vi "MultiRun Description.vi"(11 "Send Emails?":bool=TRUE) -> (3 "Send Emails? Out":bool=TRUE)   [LabVIEW 2022 SP3]
uses:
  File/Setup_Filetype.ctl
  ADAM Client/Sub VIs/ADAM Controls/Module_type_ADAM.ctl
  ADAM Client/Sub VIs/ADAM Controls/Update_scan_value.ctl
  ADAM Client/Sub VIs/ADAM Controls/Calib_type_ADAM.ctl
  ADAM Client/Sub VIs/ADAM Controls/Channel_State.ctl
  <vilib>/Utility/error.llb/Trim Whitespace One-Sided.vi
  Globals/Constants_global.vi
  Globals/Preference_global.vi
  Globals/Trav_pos_global.vi
panel:
  in  "Stop":bool
  in  "Increment Run Number":bool=TRUE
  out "Results File Prefix":string
  in  "Project":u16(ring) items=["Add New Project", "G142-3D", "G142-3D"]
  in  "OK":bool
  out "Channel Name":string
  in  "Previous Messages:":u16(ring) items=["test"]
  in  "Please add a Multi Run Description:":string
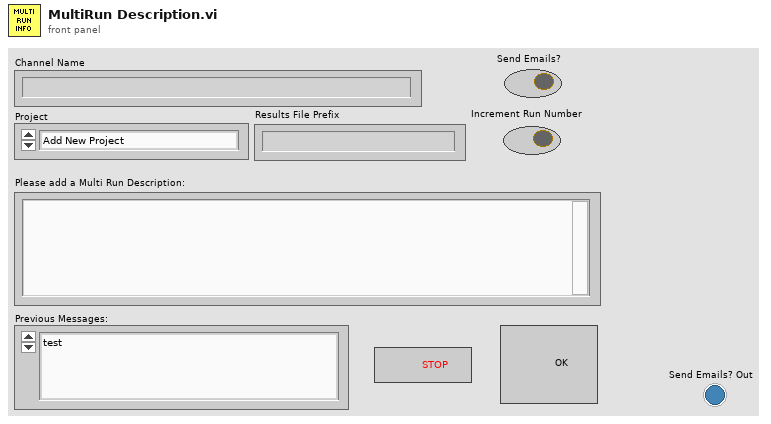
[diagram p1: front panel]
types:
  T1 = typedef "Setup_Filetype.ctl" = enum16{"Measurement Setups", "Calibration Setups", "General", "Results File Plotter Setups", "Speed Calib Tweaks"}
  T2 = typedef "Channel_State.ctl" = enum16{"On", "Off", "Always On", "Always Off"}
  T3 = typedef "Update_scan_value.ctl" = cluster{"Channel Name":string, "New Value":dbl, "!Auto_Off":bool}
  T4 = typedef "Module_type_ADAM.ctl" = string
  T5 = typedef "Ch_description_ADAM.ctl" = cluster{"Ch Name":string, "Type":T4, "Function":T6, "Ch State":T2, "Calibration type":T7, "A":dbl, "B":dbl, "C":dbl, "D":dbl, "Comments":string, "Address":T8, "String":string, "Duty":u16}
  T6 = typedef "Function_ADAM.ctl" = enum16{"Analogue Input", "Digital Input", "Event counter", "Event rate", "Analogue Output", "Digital Output", "Relay Output"}
  T7 = typedef "Calib_type_ADAM.ctl" = string
  T8 = typedef "Address.ctl" = cluster{"Main":i32, "Ch.":i32, "Sub":i32, "Port Name":string}
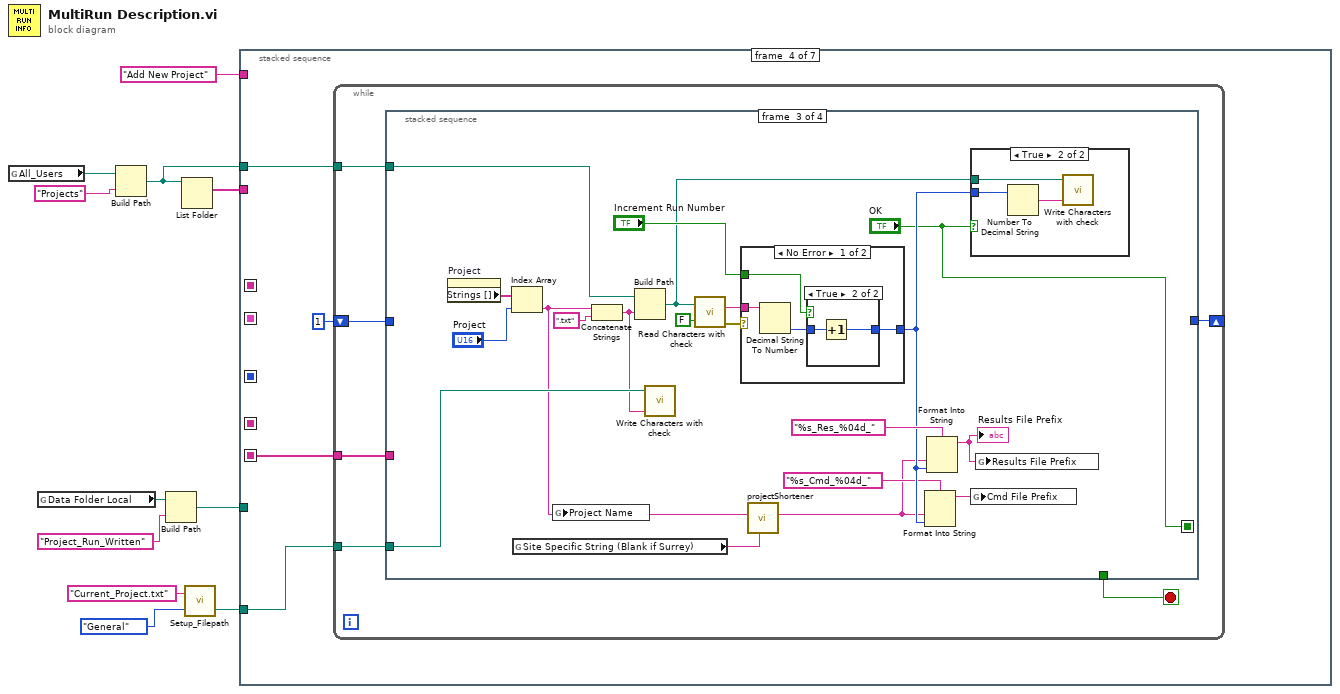
[diagram p0: block diagram]
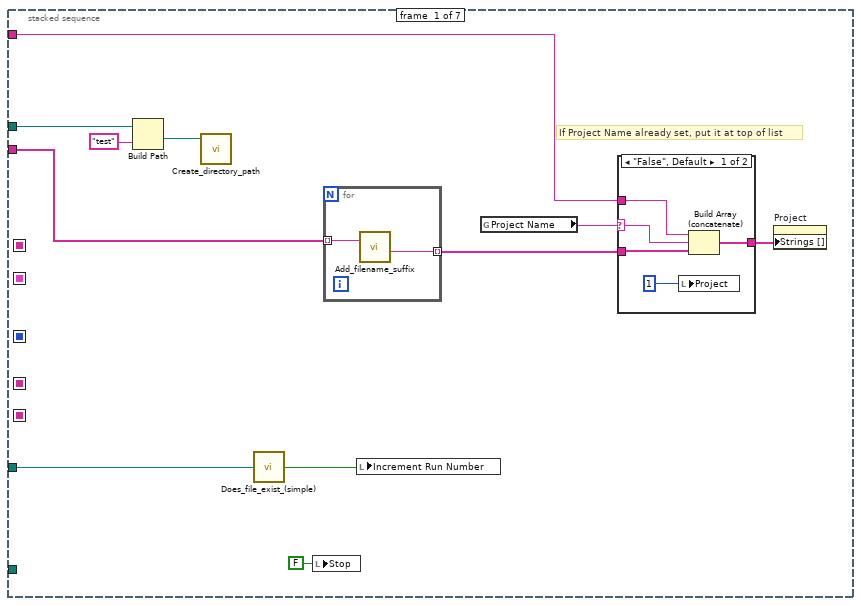
[diagram p2: hidden frame]
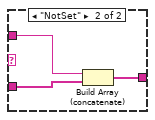
[diagram p3: hidden frame]
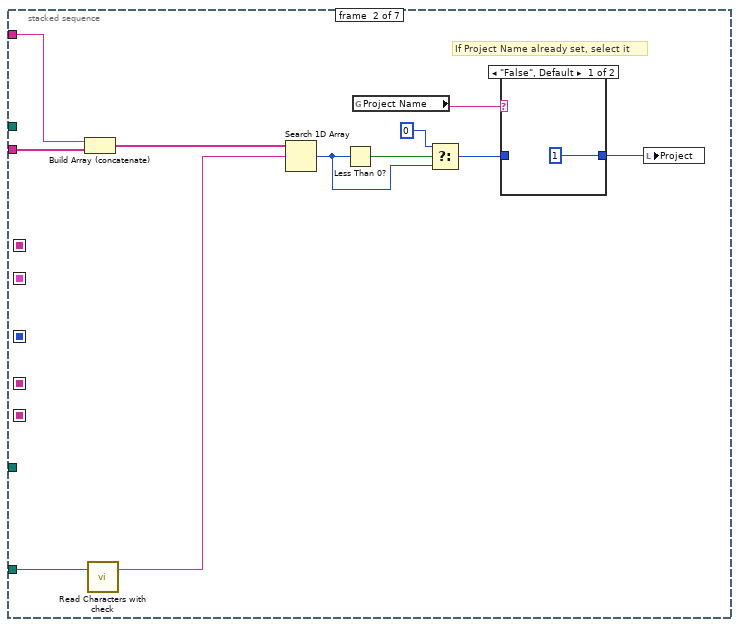
[diagram p4: hidden frame]
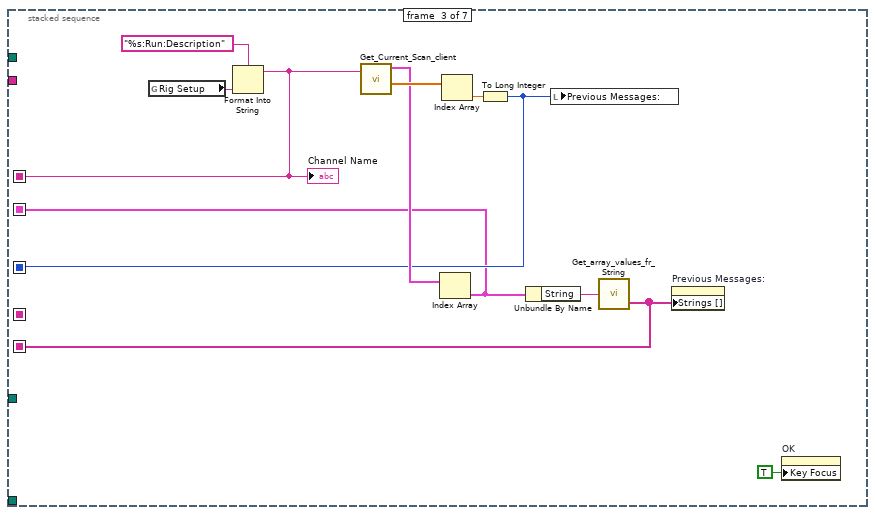
[diagram p6: hidden frame]
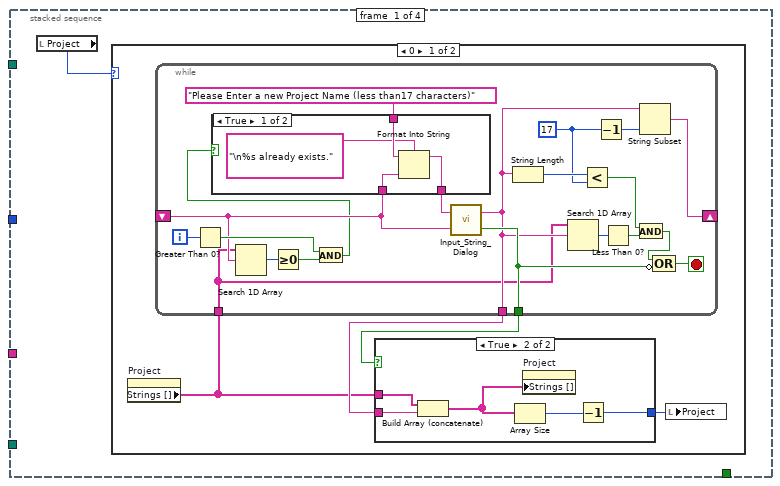
[diagram p7: hidden frame]
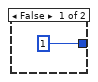
[diagram p8: hidden frame]
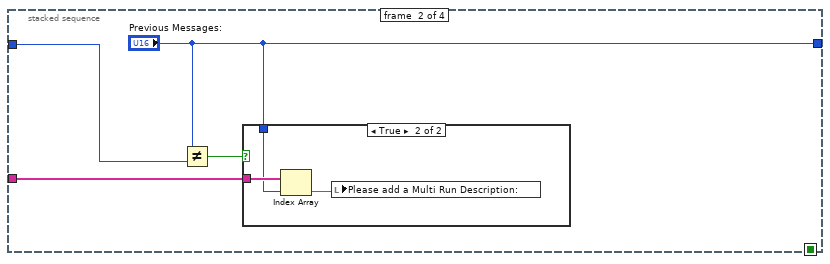
[diagram p11: hidden frame]
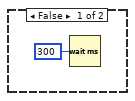
[diagram p12: hidden frame]
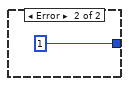
[diagram p15: hidden frame]
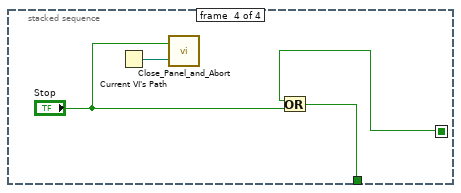
[diagram p16: hidden frame]
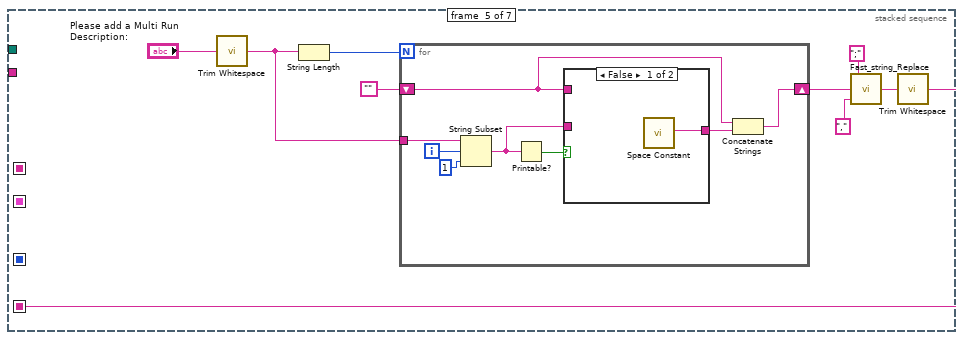
[diagram p17: hidden frame]
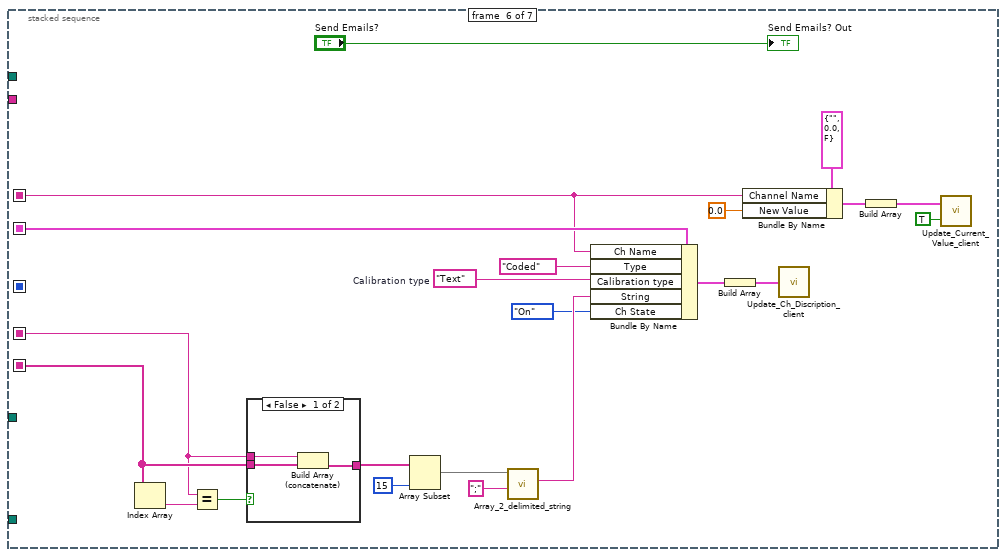
[diagram p19: hidden frame]
diagram:
  n1 = global read "Constants_global.vi" "All_Users"() -> (w8:path)
  n2 = global read "Constants_global.vi" "Data Folder Local"() -> (w3:path)
  n3 = Build Path(base path=w8, name or relative path="Projects") -> (appended path=w5:path)
  n4 = Build Path(base path=w3, name or relative path="Project_Run_Written") -> (appended path=w1:path)
  n5 = List Folder(path=w5) -> (filenames=w6:string[])  [unwired: 3 in, 3 out]
  n6 = call "Setup_Filepath.vi"("Setup File Type"=Setup_Filetype."General", "Filename in"="Current_Project.txt") -> ("Filename Out"=w9:path)  [unwired: 1 out]
  n7 = stacked-sequence {
    seq-local: [_ _ w51 _ _ _ _] -> [_ _ _ w60 _ w174 _]
    seq-local: [_ _ w49 _ _ _ _] -> [_ _ _ _ _ _ _]
    seq-local: [_ _ w48 _ _ _ _] -> [_ _ _ _ _ w186 _]
    seq-local: [_ _ w47 _ _ _ _] -> [_ _ _ _ _ w178 _]
    seq-local: [_ _ _ _ w146 _ _] -> [_ _ _ _ _ w167 _]
    tunnel: w9 -> [_ w34 _ w57 _ _ _]
    tunnel: w6 -> [w22 w40 _ _ _ _ _]
    tunnel: w5 -> [w20 _ _ w58 _ _ _]
    tunnel: "Add New Project" ("Base name") -> [w13 w41 _ _ _ _ _]
    tunnel: w1 -> [w15 _ _ _ _ _ w191]
    frame #0 {
      # "If Project Name already set, put it at top of list"
      n8 = Build Path(base path=w20, name or relative path="test") -> (appended path=w18:path)
      n9 = call "Create_directory_path.vi"("Path name"=w18) -> ()  [unwired: 2 in, 2 out]
      n10 = call "Does_file_exist_(simple).vi"("Pathname"=w15) -> ("exists?"=w16:bool)
      n11 = local write "Stop"(FALSE ("Stop")) -> ()
      n12 = for {
        tunnel: w22 -> [w32] mode=indexing
        tunnel: [w31] -> w21 mode=indexing
        n13 = call "Add_filename_suffix.vi"("Filename"=w32) -> ("Base name"=w31:string)  [unwired: 1 in, 3 out]
      }
      n14 = local write "Increment Run Number"(w16) -> ()
      n15 = global read "Preference_global.vi" "Project Name"() -> (w14:string)
      n16 = case shown="\"False\", Default" w14 {
        selector: w14 -> [w26 _]
        tunnel: w21 -> [w27 w30]
        tunnel: [w24 w29] -> w12
        tunnel: w13 -> [w25 w28]
        frame "False", Default {
          n17 = local write "Project"(1) -> ()
          n18 = Build Array (concatenate)(w25, w26, w27) -> (w24:string[])
        }
        frame "NotSet" {
          n19 = Build Array (concatenate)(w28, w30) -> (w29:string[])
        }
      }
      n20 = property on="Project" class="Ring (strict)"("Strings []"=w12) -> ()  [unwired: 2 in, 2 out]
    }
    frame #1 {
      # "If Project Name already set, select it"
      n21 = Build Array (concatenate)(w41, w40) -> (w39:string[])
      n22 = call "Read Characters with check.vi"("file (use dialog)"=w34) -> ("Read String"=w33:string)  [unwired: 1 in, 1 out]
      n23 = Search 1D Array(1D array=w39, element=w33) -> (index of element=w42:i32)  [unwired: 1 in]
      n24 = Less Than 0?(x=w42) -> (x < 0?=w43:bool)
      n25 = global read "Preference_global.vi" "Project Name"() -> (w38:string)
      n26 = Select(t=0, s=w43, f=w42) -> (s? t:f=w35:i32)
      n27 = case shown="\"False\", Default" w38 {
        tunnel: [1 ("t") w45] -> w36
        tunnel: w35 -> [_ w45]
        frame "False", Default {
        }
        frame "NotSet" {
        }
      }
      n28 = local write "Project"(w36) -> ()
    }
    frame #2 {
      n29 = global read "Preference_global.vi" "Rig Setup"() -> (w56:string)
      n30 = Format Into String(format string="%s:Run:Description", w56) -> (resulting string=w47:string)  [unwired: 2 in, 1 out]
      "Channel Name" <- w47
      n31 = call "Get_Current_Scan_client.vi"("singleChannel"=w47) -> ("Ch Description Array"=w53:T5[], "Numerical Values"=w54:dbl[])  [unwired: 1 in, 2 out]
      n32 = Index Array(array=w53) -> (element=w48:T5)  [unwired: 1 in]
      n33 = Index Array(array=w54) -> (element=w50:dbl)  [unwired: 1 in]
      n34 = To Long Integer(number=w50) -> (32bit integer=w49:i32)
      n35 = Unbundle By Name(w48) -> ("String"=w52:string)
      n36 = local write "Previous Messages:"(w49) -> ()
      n37 = call "Get_array_values_fr_String.vi"("String Value"=w52) -> ("String array"=w51:string[])  [unwired: 1 out]
      n38 = property on="Previous Messages:" class="Ring (strict)"("Strings []"=w51) -> ()  [unwired: 2 in, 2 out]
      n39 = property on="OK" class="Bool"("Key Focus"=TRUE) -> ()  [unwired: 2 in, 2 out]
    }
    frame #3 {
      n40 = while {
        shift-right: [w64] -> _
        shift-left: u16 1 ("Previous Messages") -> [w66]
        tunnel: w60 -> [w65]
        tunnel: w58 -> [w62]
        tunnel: w57 -> [w61]
        stop <- w63 stop-if-true
        n41 = stacked-sequence {
          seq-local: [_ _ "OK" _] -> [_ _ _ w145]
          tunnel: w66 -> [_ w106 _ _]
          tunnel: w65 -> [_ w104 _ _]
          tunnel: [_ "Previous Messages:" _ _] -> w64
          tunnel: [_ _ _ w144] -> w63
          tunnel: w62 -> [_ _ w126 _]
          tunnel: w61 -> [_ _ w115 _]
          frame #0 {
            n42 = local read "Project"() -> (w67:u16)
            n43 = case shown="0" w67 {
              frame 0 {
                n44 = property on="Project" class="Ring (strict)"() -> ("Strings []"=w70:string[])  [unwired: 2 in, 2 out]
                n45 = while {
                  shift-right: [w94] -> _
                  shift-left: _ -> [w88]
                  tunnel: [w84] -> w71
                  tunnel: w70 -> [w83]
                  tunnel: [w87] -> w69
                  i -> [w92]
                  stop <- w86 stop-if-true
                  w96 = 17 ("y")
                  n46 = Greater Than 0?(x=w92) -> (x > 0?=w90:bool)
                  n47 = Search 1D Array(1D array=w83, element=w88) -> (index of element=w93:i32)  [unwired: 1 in]
                  n48 = Greater Or Equal To 0?(x=w93) -> (x >= 0?=w91:bool)
                  n49 = And(x=w90, y=w91) -> (x .and. y?=w78:bool)
                  n50 = case shown="True" w78 {
                    tunnel: "Please Enter a new Project Name (less than17 characters)" ("Message to user") -> [w101 w102]
                    tunnel: w88 -> [w100 _]
                    tunnel: [w98 w102] -> w85
                    frame True {
                      n51 = Format Into String(format string="\n%s already exists.", initial string=w101, w100) -> (resulting string=w98:string)  [unwired: 1 in, 1 out]
                    }
                    frame False {
                    }
                  }
                  n52 = call "Input_String_Dialog.vi"("Value"=w88, "Message to user"=w85) -> ("Ok Out"=w87:bool, "Output string"=w84:string)
                  n53 = String Length(string=w84) -> (length=w97:i32)
                  n54 = Search 1D Array(1D array=w83, element=w84) -> (index of element=w81:i32)  [unwired: 1 in]
                  n55 = Less?(x=w97, y=w96) -> (x < y?=w82:bool)
                  n56 = Decrement(x=w96) -> (x-1=w95:i32)
                  n57 = Less Than 0?(x=w81) -> (x < 0?=w80:bool)
                  n58 = And(x=w82, y=w80) -> (x .and. y?=w79:bool)
                  n59 = String Subset(string=w84, length (rest)=w95) -> (substring=w94:string)  [unwired: 1 in]
                  n60 = Compound Arithmetic op=OR(w79, invert w87) -> (w86:bool)
                }
                n61 = case shown="True" w69 {
                  tunnel: w71 -> [_ w75]
                  tunnel: w70 -> [_ w74]
                  tunnel: [1 ("f") w73] -> w68
                  frame False {
                  }
                  frame True {
                    n62 = Build Array (concatenate)(w74, w75) -> (w77:string[])
                    n63 = Array Size(array=w77) -> (size(s)=w76:i32)
                    n64 = property on="Project" class="Ring (strict)"("Strings []"=w77) -> ()  [unwired: 2 in, 2 out]
                    n65 = Decrement(x=w76) -> (x-1=w73:i32)
                  }
                }
                n66 = local write "Project"(w68) -> ()
              }
              frame 1, Default {
              }
            }
          }
          frame #1 {
            n67 = Not Equal?(x="Previous Messages:", y=w106) -> (x != y?=w105:bool)
            n68 = case shown="True" w105 {
              tunnel: w104 -> [_ w109]
              tunnel: "Previous Messages:" -> [_ w108]
              frame False {
                n69 = Wait (ms)(milliseconds to wait=u32 300) -> ()  [unwired: 1 out]
              }
              frame True {
                n70 = Index Array(array=w109, index=w108) -> (element=w110:string)
                n71 = local write "Please add a Multi Run Description:"(w110) -> ()
              }
            }
          }
          frame #2 {
            n72 = property on="Project" class="Ring (strict)"() -> ("Strings []"=w129:string[])  [unwired: 2 in, 2 out]
            n73 = Index Array(array=w129, index="Project") -> (element=w113:string)
            n74 = global read "Preference_global.vi" "Site Specific String (Blank if Surrey)"() -> (w111:string)
            n75 = global write "Preference_global.vi" "Project Name"(w113) -> ()
            n76 = Concatenate Strings(w113, ".txt" ("string")) -> (w114:string)
            n77 = Build Path(base path=w126, name or relative path=w114) -> (appended path=w119:path)
            n78 = call "Write Characters with check.vi"("String to Write"=w114, "file (use dialog)"=w115) -> ()  [unwired: 2 in, 1 out]
            n79 = call "Read Characters with check.vi"("Call EnFlo Error Handler?"=FALSE, "file (use dialog)"=w119) -> ("error out"=w117:errorcluster, "Read String"=w118:string)
            n80 = case shown="No Error" w117 {
              tunnel: w118 -> [w137 _]
              tunnel: [w135 1] -> w123
              tunnel: "Increment Run Number" -> [w134 _]
              frame No Error {
                n81 = Decimal String To Number(string=w137) -> (number=w136:i32)  [unwired: 2 in, 1 out]
                n82 = case shown="True" w134 {
                  tunnel: w136 -> [w138 w140]
                  tunnel: [w138 w139] -> w135
                  frame False {
                  }
                  frame True {
                    n83 = Increment(x=w140) -> (x+1=w139:i32)
                  }
                }
              }
              frame Error {
              }
            }
            n84 = call "projectShortener.vi"("Site Specific String (Blank if Surrey)"=w111, "fullProjectName"=w113) -> ("projectNameOut"=w112:string)  [unwired: 9 in]
            n85 = Format Into String(format string="%s_Cmd_%04d_", w112, w123) -> (resulting string=w121:string)  [unwired: 2 in, 1 out]
            n86 = Format Into String(format string="%s_Res_%04d_", w112, w123) -> (resulting string=w125:string)  [unwired: 2 in, 1 out]
            "Results File Prefix" <- w125
            n87 = case shown="True" "OK" {
              tunnel: w119 -> [_ w132]
              tunnel: w123 -> [_ w133]
              frame False {
              }
              frame True {
                n88 = Number To Decimal String(number=w133) -> (decimal integer string=w131:string)  [unwired: 1 in]
                n89 = call "Write Characters with check.vi"("String to Write"=w131, "file (use dialog)"=w132) -> ()  [unwired: 2 in, 1 out]
              }
            }
            n90 = global write "Trav_pos_global.vi" "Cmd File Prefix"(w121) -> ()
            n91 = global write "Trav_pos_global.vi" "Results File Prefix"(w125) -> ()
          }
          frame #3 {
            n92 = Current VI's Path() -> (path=w143:path)
            n93 = call "Close_Panel_and_Abort.vi"("Vi path"=w143, "stop"="Stop") -> ()  [unwired: 1 out]
            n94 = Or(x=w145, y="Stop") -> (x .or. y?=w144:bool)
          }
        }
      }
    }
    frame #4 {
      n95 = call <vilib>:"Trim Whitespace.vi"("string"="Please add a Multi Run Description:") -> ("trimmed string"=w151:string)  [unwired: 1 in]
      n96 = String Length(string=w151) -> (length=w150:i32)
      n97 = for {
        N: w150 -> [_]
        shift-right: [w156] -> w149
        shift-left: "" -> [w157]
        tunnel: w151 -> [w160]
        i -> [w161]
        n98 = String Subset(string=w160, offset (0)=w161, length (rest)=1 ("length (rest)")) -> (substring=w158:string)
        n99 = Printable?(1:w158) -> (0:w159:bool)
        n100 = case shown="False" w159 {
          tunnel: w157 -> [_ _]
          tunnel: w158 -> [_ w164]
          tunnel: [w163 w164] -> w155
          frame False {
            n101 = call <vilib>:"Space Constant.vi"() -> ("String"=w163:string)
          }
          frame True {
          }
        }
        n102 = Concatenate Strings(w157, w155) -> (w156:string)
      }
      n103 = call "Fast_string_Replace.vi"("Replace match with:"=",", "Input String"=w149, "matchThis"=";" ("regular expression")) -> ("Output String"=w147:string)  [unwired: 1 in, 1 out]
      n104 = call <vilib>:"Trim Whitespace.vi"("string"=w147) -> ("trimmed string"=w146:string)  [unwired: 1 in]
    }
    frame #5 {
      w168 = T7 "Text"  # Calibration type
      n105 = Index Array(array=w174) -> (element=w173:string)  [unwired: 1 in]
      n106 = Equal?(x=w167, y=w173) -> (x = y?=w172:bool)
      n107 = case shown="False" w172 {
        tunnel: [w189 w190] -> w171
        tunnel: w174 -> [w188 w190]
        tunnel: w167 -> [w187 _]
        frame False {
          n108 = Build Array (concatenate)(w187, w188) -> (w189:string[])
        }
        frame True {
        }
      }
      n109 = Array Subset(array=w171, length=15) -> (w170:string[])  [unwired: 1 in]
      n110 = call "Array_2_delimited_string.vi"("delimiter (Tab)"=";", "Array of Strings"=w170) -> ("delimited string"=w183:string)  [unwired: 9 in]
      n111 = Bundle By Name(cluster=w186, "Ch Name"=w178, "Type"=T4 "Coded", "Calibration type"=w168, "String"=w183, "Ch State"=Channel_State."On") -> (w182:T5)
      n112 = Build Array(w182) -> (w181:T5[])
      n113 = Bundle By Name(cluster=T3 {"Channel Name"="", "New Value"=0.0, "!Auto_Off"=FALSE} ("Update Scan Value Cluster"), "Channel Name"=w178, "New Value"=0.0) -> (w176:T3)
      n114 = call "Update_Ch_Discription_client.vi"("Channels to update In"=w181) -> ()  [unwired: 1 in]
      n115 = Build Array(w176) -> (w175:T3[])
      n116 = call "Update_Current_Value_client.vi"("Don't Bother with check?"=TRUE, "Update array in"=w175) -> ()
      "Send Emails? Out" <- "Send Emails?"
    }
    frame #6 {
      n117 = local read "Increment Run Number"() -> (w192:bool)
      n118 = case shown="True" w192 {
        tunnel: w191 -> [_ w193]
        frame False {
        }
        frame True {
          n119 = Delete(path (use dialog)=w193) -> ()  [unwired: 4 in, 3 out]
        }
      }
    }
  }
